vi "Launch Installer Helper.vi"(7 "Listbox Ref":refnum<vi>, 8 "Error In":errorcluster, 9 "Dep Index":i32, 10 "File Path Control":path, 11 "Dependecy Config":T1) -> (0 "Error Out":errorcluster)   [LabVIEW 2011, in "LMH-Toolbox.lvlib" / "LMH-Installer Tools.lvlib"]
uses:
  LMH-Installer Tools.lvlib
  Type Defs/Dependency Config.ctl
  Type Defs/Dependecy.ctl
  Common/Private/Web/Type Defs/Download Task.ctl
  Common/LMH-Common.lvlib
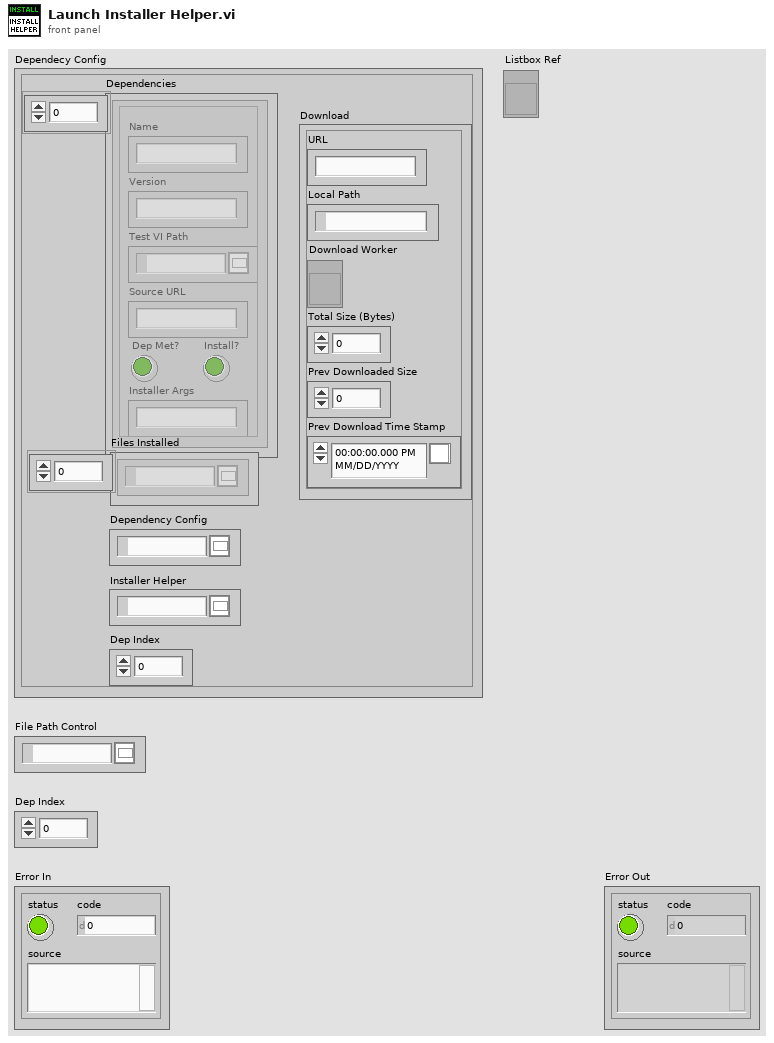
[diagram p1: front panel]
types:
  T1 = typedef "LMH-Toolbox.lvlib/LMH-Installer Tools.lvlib/Dependency Config.ctl" = cluster{"Dependencies":T2[], "Files Installed":path[], "Dependency Config":path, "Installer Helper":path, "Dep Index":i32, "Download":T3}
  T2 = typedef "LMH-Toolbox.lvlib/LMH-Installer Tools.lvlib/Dependecy.ctl" = cluster{"Name":string, "Version":string, "Test VI Path":path, "Source URL":string, "Dep Met?":bool, "Install?":bool, "Installer Args":string}
  T3 = typedef "LMH-Toolbox.lvlib/LMH-Common.lvlib/Download Task.ctl" = cluster{"URL":string, "Local Path":path, "Download Worker":refnum<vi>, "Total Size (Bytes)":u64, "Prev Downloaded Size":u64, "Prev Download Time Stamp":timestamp}
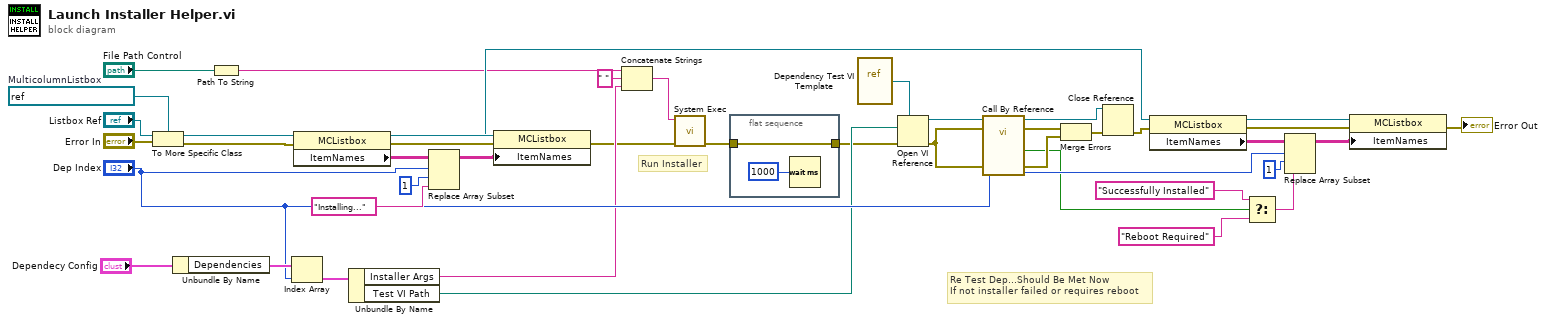
[diagram p0: block diagram]
diagram:
  w41 = refnum<vi> refnum  # MulticolumnListbox
  # "Re Test Dep...Should Be Met Now\nIf not installer failed or requires reboot"
  # "Run Installer"
  n1 = To More Specific Class(target class=w41, reference="Listbox Ref", error in="Error In") -> (specific class reference=w27:refnum<vi>, error out=w26:errorcluster)
  n2 = Unbundle By Name("Dependecy Config") -> ("Dependencies"=w23:T2[])
  n3 = Path To String(path="File Path Control") -> (string=w18:string)
  n4 = Index Array(array=w23, index="Dep Index") -> (element=w21:T2)
  n5 = property class="MCListbox"(reference=w27, error in=w26) -> (reference out=w29:refnum<vi>, error out=w30:errorcluster, "ItemNames"=w31:string[][])
  n6 = Unbundle By Name(w21) -> ("Installer Args"=w17:string, "Test VI Path"=w9:path)
  n7 = Replace Array Subset(array=w31, new element="Installing..." ("new element/subarray"), index (row)="Dep Index", index (col)=1 ("disabled index (col)")) -> (w32:string[][])
  n8 = property class="MCListbox"(reference=w29, error in=w30, "ItemNames"=w32) -> (reference out=w28:refnum<vi>, error out=w3:errorcluster)
  n9 = Concatenate Strings(w18, " " ("string"), w17) -> (w19:string)
  n10 = call <vilib>:"System Exec.vi"("error in (no error)"=w3, "command line"=w19) -> ("error out"=w2:errorcluster)  [unwired: 6 in, 3 out]
  n11 = flat-sequence {
    tunnel: w2 -> [w44]
    tunnel: [w44] -> w1
    frame #0 {
      n12 = Wait (ms)(milliseconds to wait=u32 1000) -> ()  [unwired: 1 out]
    }
  }
  n13 = vi-ref "Dependency Test VI Template.vi"() -> (w15:refnum<vi>)
  n14 = Open VI Reference(type specifier VI Refnum (for type only)=w15, vi path=w9, error in (no error)=w1) -> (vi reference=w16:refnum<vi>, error out=w14:errorcluster)  [unwired: 3 in]
  n15 = call-by-ref "?"(reference=w16, error in=w14, "Error In"=w14) -> (reference out=w10:refnum<vi>, error out=w13:errorcluster, "Error Out"=w12:errorcluster, "Pass?"=w7:bool)  [unwired: 9 in]
  n16 = Merge Errors(w13, w12) -> (w11:errorcluster)
  n17 = Close Reference(reference=w10, error in (no error)=w11) -> (error out=w8:errorcluster)
  n18 = property class="MCListbox"(reference=w28, error in=w8) -> (reference out=w39:refnum<vi>, error out=w38:errorcluster, "ItemNames"=w37:string[][])
  n19 = Select(t="Successfully Installed" ("new element/subarray"), s=w7, f="Reboot Required" ("new element/subarray")) -> (s? t:f=w4:string)
  n20 = Replace Array Subset(array=w37, new element=w4, index (row)="Dep Index", index (col)=1 ("disabled index (col)")) -> (w36:string[][])
  n21 = property class="MCListbox"(reference=w39, error in=w38, "ItemNames"=w36) -> (error out=→"Error Out":errorcluster)  [unwired: 1 out]
